vi "VISnipDirectory.vi"(8 "error in (no error)":errorcluster, 10 "Parameters":string[](array[string])) -> (0 "error out":errorcluster)   [LabVIEW 2013]
panel:
  # "VI Root"
  # "PNG Root"
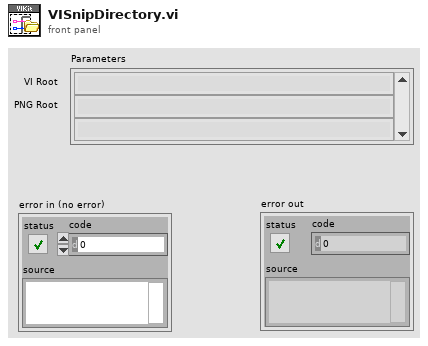
[diagram p1: front panel]
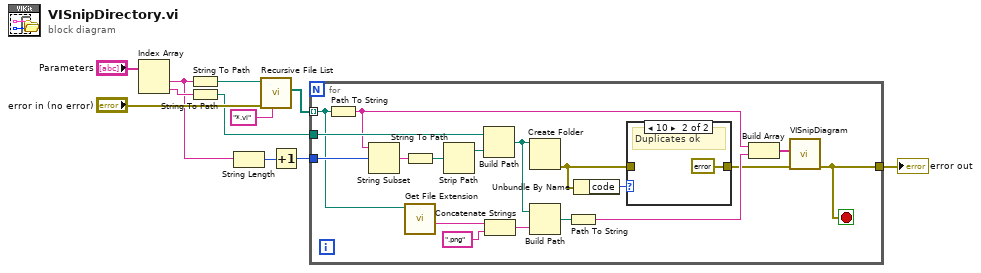
[diagram p0: block diagram]
diagram:
  n1 = Index Array(array="Parameters") -> (element #1=w5:string, element #2=w10:string)  [unwired: 2 in]
  n2 = String To Path(string=w5) -> (path=w9:path)
  n3 = String To Path(string=w10) -> (path=w2:path)
  n4 = String Length(string=w5) -> (length=w6:i32)
  n5 = call <vilib>:"Recursive File List.vi"("pattern"="*.vi", "error in (no error)"="error in (no error)", "Folder Path"=w9) -> ("All Files in Dir"=w4:path[])  [unwired: 4 in, 4 out]
  n6 = Increment(x=w6) -> (x+1=w3:i32)
  n7 = for {
    tunnel: w3 -> [w29]
    tunnel: w4 -> [w24] mode=indexing
    tunnel: w2 -> [w25]
    tunnel: [w15] -> w1
    stop <- w15 stop-if-true
    n8 = Path To String(path=w24) -> (string=w16:string)
    n9 = String Subset(string=w16, offset (0)=w29) -> (substring=w28:string)  [unwired: 1 in]
    n10 = String To Path(string=w28) -> (path=w27:path)
    n11 = call <vilib>:"Get File Extension.vi"("file"=w24) -> ("filename without extension"=w23:string)  [unwired: 7 in, 3 out]
    n12 = Strip Path(path=w27) -> (stripped path=w26:path)  [unwired: 1 out]
    n13 = Build Path(base path=w25, name or relative path=w26) -> (appended path=w20:path)
    n14 = Concatenate Strings(w23, ".png" ("string")) -> (w21:string)
    n15 = Create Folder(path (use dialog)=w20) -> (error out=w13:errorcluster)  [unwired: 2 in, 2 out]
    n16 = Build Path(base path=w20, name or relative path=w21) -> (appended path=w19:path)
    n17 = Path To String(path=w19) -> (string=w18:string)
    n18 = Unbundle By Name(w13) -> ("code"=w14:i32)
    n19 = case shown="10" w14 {
      tunnel: w13 -> [w30 _]
      tunnel: [w30 errorcluster {"status"=FALSE, "code"=0, "source"=""} ("error out")] -> w12
      frame 0, Default {
      }
      frame 10 {
        # "Duplicates ok"
      }
    }
    n20 = Build Array(w16, w18) -> (w17:string[])
    n21 = call "VISnipDiagram.vi"("error in (no error)"=w12, "Parameters"=w17) -> ("error out"=w15:errorcluster)  [unwired: 9 in]
  }
  "error out" <- w1
